vi "BytesAtSerialPort.vi"(8 "error in (no error)":errorcluster, 11 "VISA Refnum in":T1) -> (0 "error out":errorcluster, 2 "Bytes at Port":u32, 3 "VISA Refnum in":T1)   [LabVIEW 2020]
uses:
  SerialCtrl.ctl
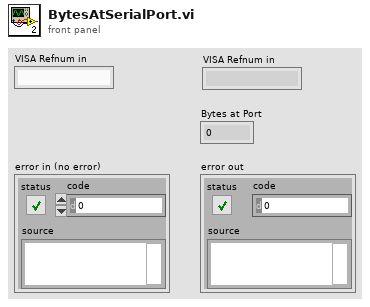
[diagram p1: front panel]
types:
  T1 = typedef "SerialCtrl.ctl" = string
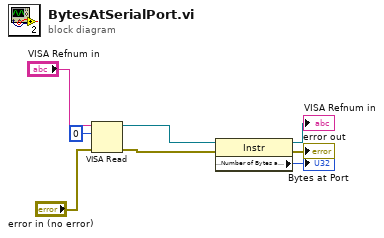
[diagram p0: block diagram]
diagram:
  n1 = VISA Read(VISA resource name="VISA Refnum in", byte count=u32 0, error in (no error)="error in (no error)") -> (VISA resource name out=w4:refnum<visa-resource-name>, error out=w2:errorcluster)  [unwired: 2 out]
  n2 = property class="Instr"(reference=w4, error in=w2) -> (reference out=→"VISA Refnum in":refnum<visa-resource-name>, error out=→"error out":errorcluster, "Serial Settings:Number of Bytes at Serial Port"=→"Bytes at Port":u32)
